vi "drive_test_load_allmat_hyst_sat.vi"() -> ()   [LabVIEW 2017]
uses:
  <vilib>/Analysis/Matrix/Datatypes/RealMatrix.ctl
  <vilib>/userdefined/High Color/nirio_resource_hc.ctl
  <vilib>/FPGAPlugInAG/cRIO-9082/niLvFpga_Open_cRIO-9082.vi
  <vilib>/rvi/interface/common/dynamic/niFpgaDynamicAddResources.vi
  <vilib>/FPGAPlugInAG/Dynamic/niLvFpga_Reset_Dynamic.vi
  <vilib>/rvi/interface/common/niFpgaWaitOnOcc.vi
  <vilib>/Utility/error.llb/Error Cluster From Error Code.vi
  <vilib>/rvi/errors/niLvFpgaAdjustHostInterfaceError.vi
  <vilib>/FPGAPlugInAG/Dynamic/niLvFpga_Run_Dynamic.vi
  <vilib>/rvi/interface/nirviOpenFPGA/nirviOpenFPGA.xnode
  FPGA Bitfiles/afmimagingcontro_FPGATargetSPARTA_testloadallmathy_0qXaUSwVF44.lvbitx
  <vilib>/rvi/interface/nirviMethod/nirviMethod.xnode
  <vilib>/rvi/interface/nirviReadWriteControl/nirviReadWriteControl.xnode
  <vilib>/rvi/errors/niLvFpgaMergeErrorWithErrorCode.vi
  <vilib>/rvi/interface/Simulation/niFpgaSimulationCallBeginRW.vi
  NiFpgaLv.dll
  <vilib>/FPGAPlugInAG/Dynamic/niLvFpga_ConfigureFifo_Dynamic.vi
  <vilib>/FPGAPlugInAG/Dynamic/niLvFpga_WriteFifo_Dynamic.vi
  <vilib>/Analysis/Matrix/NI_Matrix.lvlib
panel:
  out "x-y":u32
  out "Actual Depth":u32
  out "Empty Elements Remaining":u32
  out "AllMatrix":dbl[](array[numeric])
  out "Ns_obs/cntrl":u8
  in  "sat_ws":T1=[[0.0068, -0.0396, -0.0381, 0.7363, 0.0459, 0.0728, 0.0723]]
  in  "sat_ds":T1=[[-9.0, -5.399, -1.7998, 0.0, 1.7998, 5.3999, 9.0]]
  in  "N_sat":i32
  in  "N_hyst":i32
  in  "w_s":T1=[[1.3794, -0.2251, -0.103, -0.0527, -0.04, -0.0327, -0.0591]]
  in  "r_s":T1
  in  "Tab Control":T2(tab)
  out "AllMatHS Length":i32
  in  "control_data_path":path=path "Z:/mpc-journal/step-exps/FXP_lin_Controls01.csv"
  in  "ABORT":bool
  out "hyst_ws":fxp<+/-,16,5>[](array[numeric])
  out "hyst_rs":fxp<+/-,16,5>[](array[numeric])
  out "sat_ws 2":fxp<+/-,16,5>[](array[numeric])
  out "sat_ds 2":fxp<+/-,16,5>[](array[numeric])
  out "SS FIFO TimeOut?":bool
  out "Array":dbl[](array[numeric])
  out "K_fxp":fxp<+/-,16,5>[](array[numeric])
  out "L_fxp":fxp<+/-,16,5>[](array[numeric])
  in  "stop":bool
  out "ControlMatrices":T3
  # "yk\nulin\ndu\nu_inv\nIpow\nX"
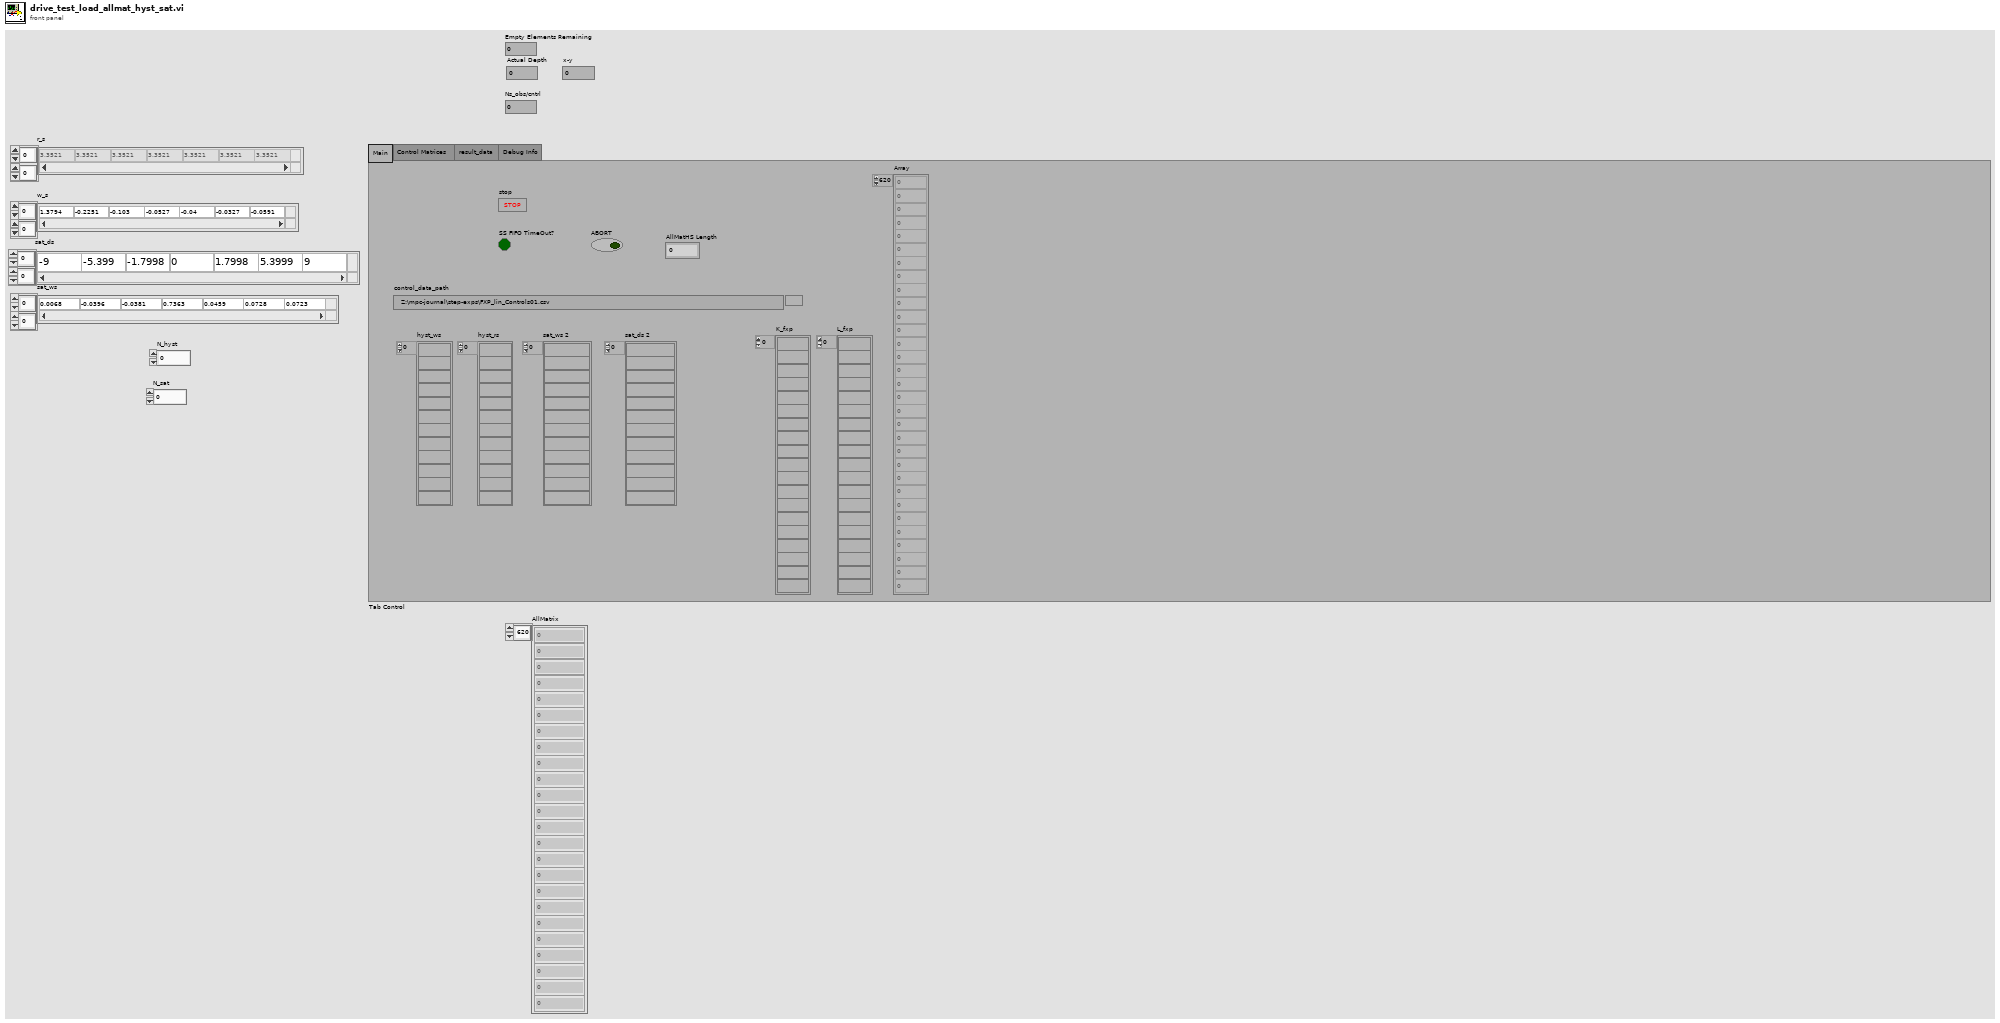
[diagram p1: front panel]
types:
  T1 = typedef "NI_Matrix.lvlib/RealMatrix.ctl" = dbl[][]
  T2 = enum32{"Main", "Control Matrices", "result_data", "Debug Info"}
  T3 = cluster{"Az":fxp<+/-,32,4>[][], "Bz":dbl[][], "Lz":dbl[][], "Kz":dbl[][], "NxNu":dbl[][]}
  T4 = typedef "nirio_resource_hc.ctl" = tag
  T5 = typedef "FXPControlParams_distEst.ctl" = cluster{"umax":fxp<+/-,18,5>, "Ns_obs/cntrl":u8, "ref_f_VEC":fxp<+/-,32,5>[], "du_max":fxp<+/-,18,5>, "Nbar":fxp<+/-,32,5>}
  T6 = typedef "ObserverMatrices.ctl" = cluster{"Az":fxp<+/-,32,4>[][], "Bz":dbl[][], "Lz":dbl[][], "Kz":dbl[][], "NxNu":dbl[][]}
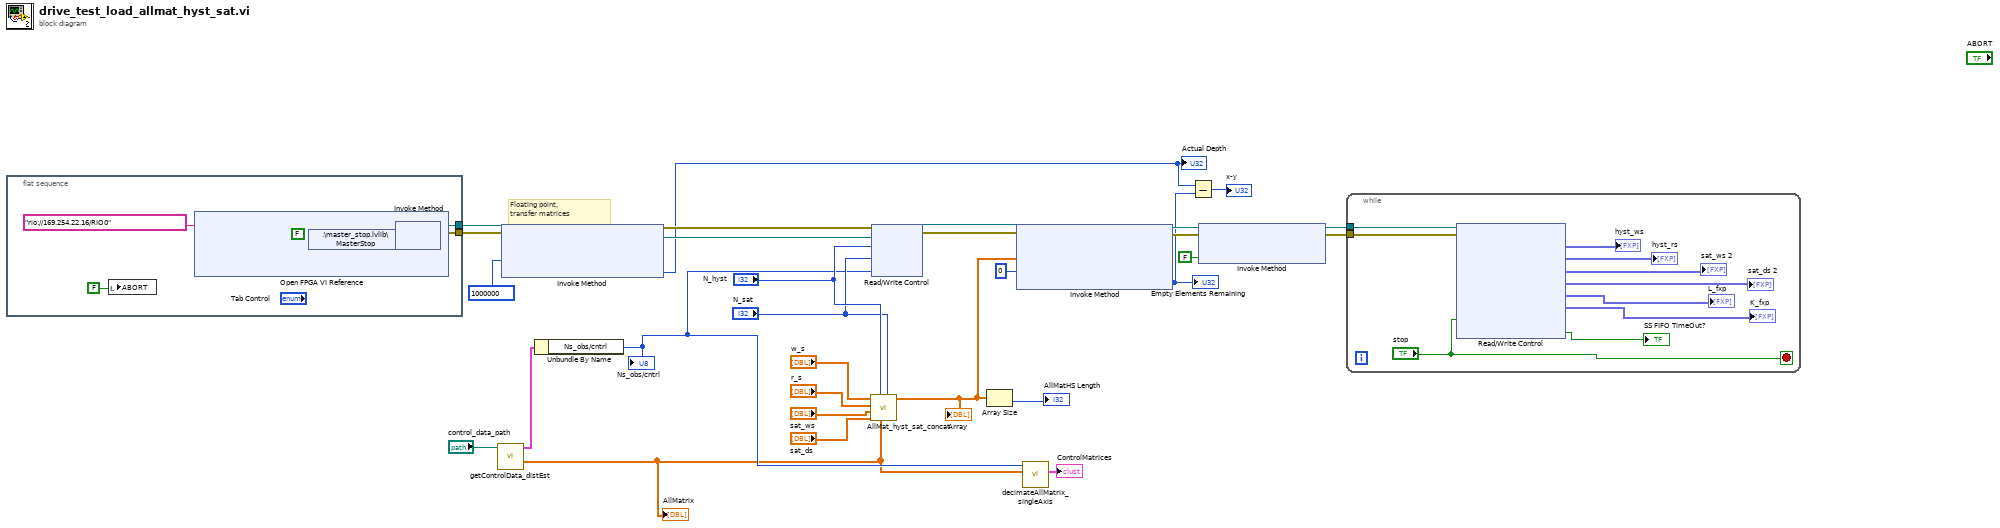
[diagram p0: block diagram]
diagram:
  # "Floating point, \ntransfer matrices"
  n1 = flat-sequence {
    tunnel: [w36] -> w26
    tunnel: [w35] -> w25
    frame #0 {
      n2 = local write "ABORT"(FALSE) -> ()
      n3 = xnode "Open FPGA VI Reference"("resource name"=T4 "rio://169.254.22.16/RIO0") -> ("FPGA VI Reference Out"=w34:refnum<k20>, "error out"=w32:errorcluster)  [unwired: 1 in]
      n4 = shared-variable ".\\master_stop.lvlib\\MasterStop"(FALSE ("MasterStop"), error in=w32) -> (error out=w33:errorcluster)
      n5 = xnode "Invoke Method"("FPGA VI Reference In"=w34, "error in"=w33) -> ("FPGA VI Reference Out"=w36:refnum<k20>, "error out"=w35:errorcluster)
    }
  }
  n6 = call "getControlData_distEst.vi"("system matricec path"="control_data_path") -> ("AllMatrix"=w4:dbl[], "ControlParams"=w23:T5)  [unwired: 8 in, 1 out]
  "AllMatrix" <- w4
  n7 = xnode "Invoke Method"("FPGA VI Reference In"=w26, "error in"=w25, "Requested Depth"=u32 1000000) -> ("FPGA VI Reference Out"=w8:refnum<k20>, "error out"=w7:errorcluster, "Actual Depth"=w3:u32)
  "Actual Depth" <- w3
  n8 = Unbundle By Name(w23) -> ("Ns_obs/cntrl"=w6:u8)
  "Ns_obs/cntrl" <- w6
  n9 = call "AllMat_hyst_sat_concat.vi"("N_sat"="N_sat", "AllMatrix"=w4, "N_hyst"="N_hyst", "sat_ds"="sat_ds", "sat_ws"="sat_ws", "r_s"="r_s", "w_s"="w_s") -> ("Array"=w19:dbl[])  [unwired: 4 in]
  "Array" <- w19
  n10 = xnode "Read/Write Control"("FPGA VI Reference In"=w8, "error in"=w7, "N_hyst"="N_hyst", "N_sat"="N_sat", "NS_O/C"=w6) -> ("FPGA VI Reference Out"=w28:refnum<k20>, "error out"=w27:errorcluster)
  n11 = Array Size(array=w19) -> (size(s)=→"AllMatHS Length":i32)
  n12 = xnode "Invoke Method"("FPGA VI Reference In"=w28, "error in"=w27, "Data"=w19, "Timeout (ms)"=0) -> ("FPGA VI Reference Out"=w13:refnum<k20>, "error out"=w12:errorcluster, "Empty Elements Remaining"=w2:u32)
  "Empty Elements Remaining" <- w2
  n13 = call "decimateAllMatrix_singleAxis.vi"("AllMatrix"=w4, "NS_obs/cntrl"=w6) -> ("ControlMatrices"=→"ControlMatrices":T6)  [unwired: 8 in, 1 out]
  n14 = Subtract(x=w3, y=w2) -> (x-y=→"x-y":u32)
  n15 = xnode "Invoke Method"("FPGA VI Reference In"=w13, "error in"=w12, "Wait Until Done (F)"=FALSE) -> ("FPGA VI Reference Out"=w10:refnum<k20>, "error out"=w9:errorcluster)
  n16 = while {
    tunnel: w10 -> [w47]
    tunnel: w9 -> [w46]
    stop <- "stop" stop-if-true
    n17 = xnode "Read/Write Control"("FPGA VI Reference In"=w47, "error in"=w46, "stop"="stop") -> ("hyst_ws"=→"hyst_ws":fxp<+/-,16,5>[], "hyst_rs"=→"hyst_rs":fxp<+/-,16,5>[], "sat_ws"=→"sat_ws 2":fxp<+/-,16,5>[], "sat_ds"=→"sat_ds 2":fxp<+/-,16,5>[], "L_fxp"=→"L_fxp":fxp<+/-,16,5>[], "K_fxp"=→"K_fxp":fxp<+/-,16,5>[], "SS FIFO TimeOut?"=→"SS FIFO TimeOut?":bool)  [unwired: 2 out]
  }
